vi "ChangeLight.vi"(0 "object in":refnum<class "RedState.lvclass">, 5 "Error In":errorcluster) -> (14 "object out":refnum<class "State.lvclass">, 19 "Error Out":errorcluster)   [LabVIEW 2024, in "RedState.lvclass"]
uses:
  RedState.lvclass
  State_interface/State.lvclass
  YellowState_class/YellowState.lvclass
  C:/Users/burakkorkmaz/Desktop/Leveling/labview-desing-patterns/State Pattern/State_interface/State.lvclass
  RedState.lvclass/RedState.ctl
panel:
  # "Connector Pane"
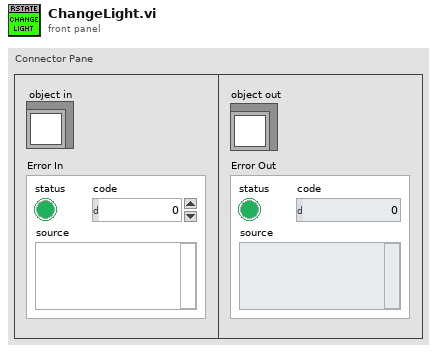
[diagram p1: front panel]
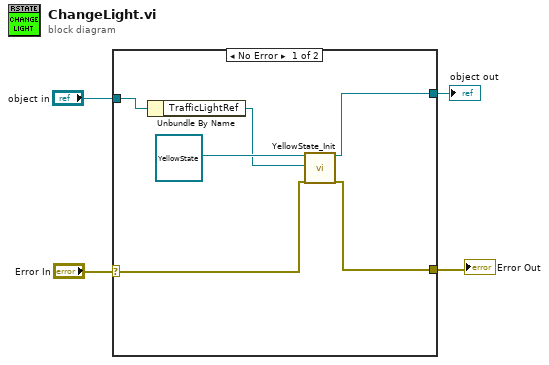
[diagram p0: block diagram]
diagram:
  n1 = case shown="No Error" "Error In" {
    selector: "Error In" -> [w7 w11]
    tunnel: [w8 w11] -> w3
    tunnel: "object in" -> [w10 _]
    tunnel: [w5 _] -> w1
    frame No Error {
      n2 = Unbundle By Name(w10) -> ("TrafficLightRef"=w6:refnum<class "TrafficLight.lvclass">)
      n3 = call "YellowState_Init.vi"("object in"=refnum<class "YellowState.lvclass"> refnum ("YellowState"), "TrafficLight"=w6, "Error In"=w7) -> ("object out"=w5:refnum<class "YellowState.lvclass">, "Error Out"=w8:errorcluster)  [unwired: 15 in]
    }
    frame Error {
    }
  }
  "Error Out" <- w3
  "object out" <- w1
